vi "Report Options.vi"(5 "LensList":i32[](array[numeric]), 6 "Search Window":dbl=3.0 min=0.1 format="%#.6f", 7 "Min. Height":dbl=1.0 min=1.0 format="%#.6f", 8 "Min. Width":i32=4 min=2 max=100, 9 "RefMass":dbl[](array[numeric])) -> (0 "Search Window 2":dbl=3.0 min=0.1 format="%#.6f", 1 "Min. Height 2":dbl=1.0 min=1.0 format="%#.6f", 2 "Min. Width 2":i32=4 min=2 max=100, 3 "RefMass 2":dbl[](array[numeric]), 4 "LensList 2":i32[](array[numeric]))   [LabVIEW 2012]
uses:
  Configuration/_Global Configuration.vi
  <vilib>/Utility/file.llb/Read From Spreadsheet File (DBL).vi
  <vilib>/Utility/file.llb/Write To Spreadsheet File (DBL).vi
  <vilib>/Utility/config.llb/Write Key (String).vi
  <vilib>/Utility/config.llb/Write Key (Double).vi
  <vilib>/Utility/config.llb/Write Key (I32).vi
  <vilib>/Utility/config.llb/NI_LVConfig.lvlib
panel:
  in  "Tab Control":enum32{"Lens Selection", "Peak List Options"}(tab)
  in  "Delete":bool
  in  "Insert":bool
  in  "Current Lens":u16(ring)
  in  "Lens Values":i32(listbox)
  in  "Save":bool
  in  "Load":bool
  in  "Current Reference":dbl=500.0 min=0.0 max=3000.0 format="%#.2f"
  in  "Insert 2":bool
  in  "Delete 2":bool
  in  "Mass Reference (amu)":i32(listbox)
  # "Peak Parameter"
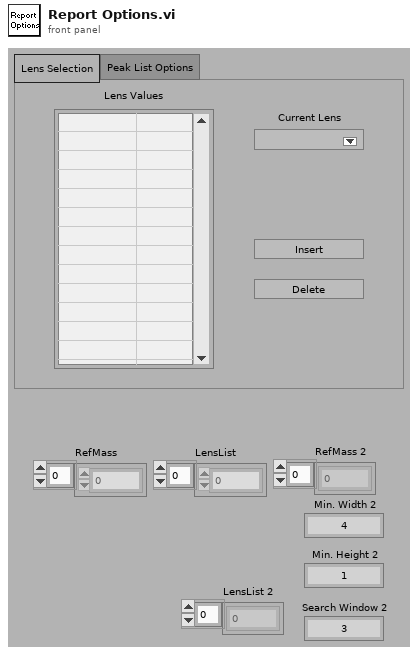
[diagram p1: front panel]
types:
  T1 = enum32{"existing file", "new file", "new or existing file", "existing dir", "new dir", "new or existing dir", "existing file (use LLBs)", "new file (use LLBs)", "new or existing file (use LLBs)", "new or existing file or directory (use LLBs)"}
  T2 = typedef "_RT Instrument 2.ctl" = cluster{"Table":T3[], "Instrument":string[]}
  T3 = typedef "_RT Configuration 2.ctl" = cluster{"Name":string, "Ch#":u8, "Min":dbl, "Max":dbl, "Def+":dbl, "Def-":dbl, "Offset":dbl, "Slope":dbl, "Type":u8, "Description":string, "SettleT":dbl}
  T4 = typedef "NI_LVConfig.lvlib/Config Data RefNum.ctl" = refnum<k1>
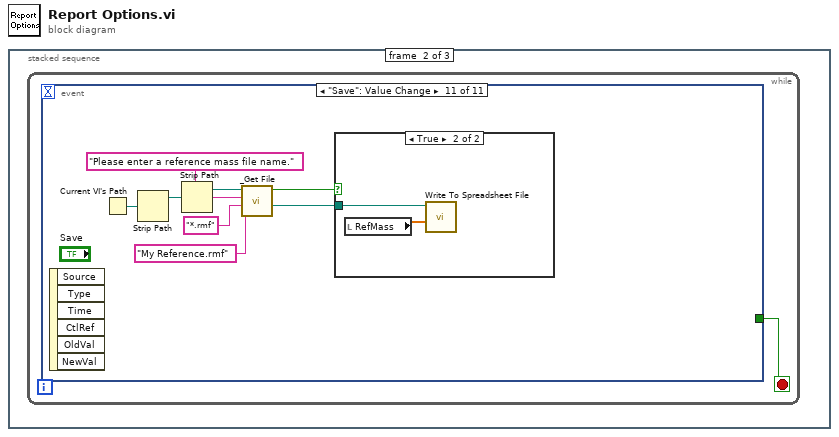
[diagram p0: block diagram]
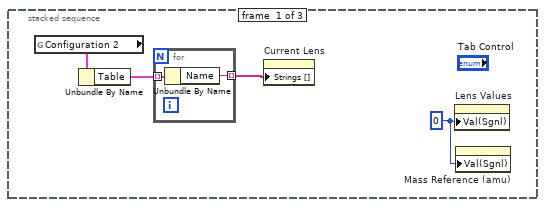
[diagram p2: hidden frame]
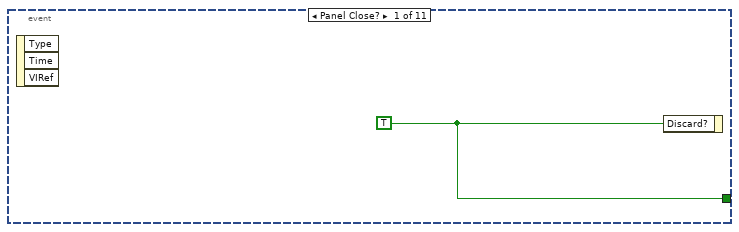
[diagram p3: hidden frame]
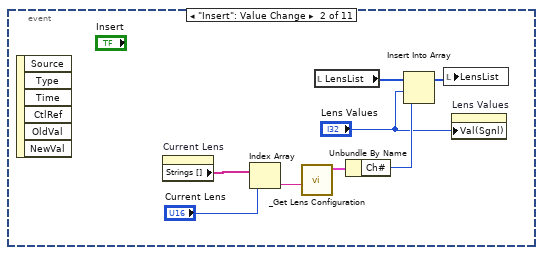
[diagram p4: hidden frame]
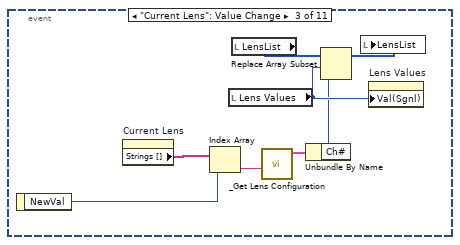
[diagram p5: hidden frame]
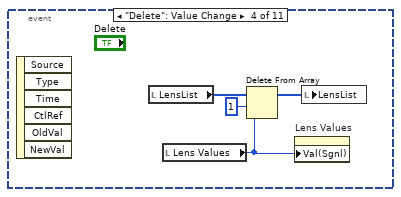
[diagram p6: hidden frame]
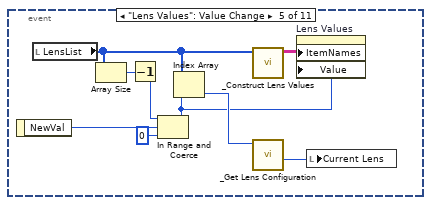
[diagram p7: hidden frame]
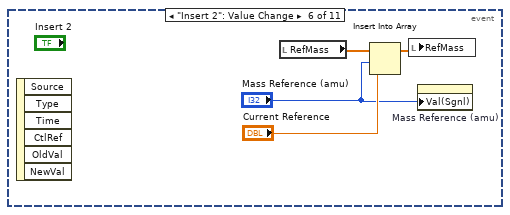
[diagram p8: hidden frame]
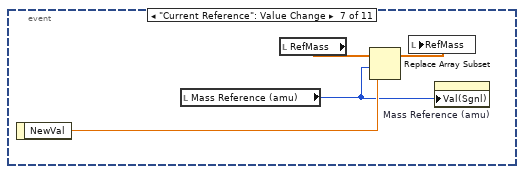
[diagram p9: hidden frame]
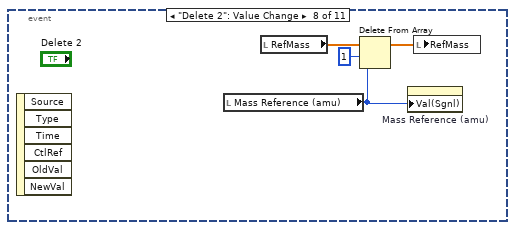
[diagram p10: hidden frame]
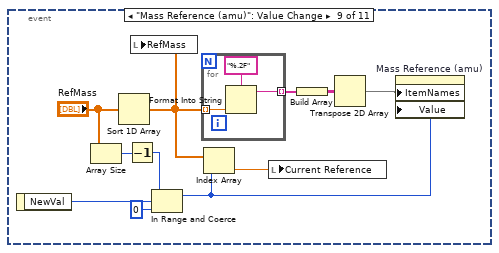
[diagram p11: hidden frame]
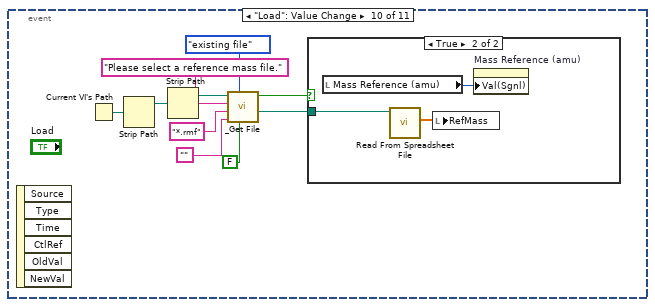
[diagram p12: hidden frame]
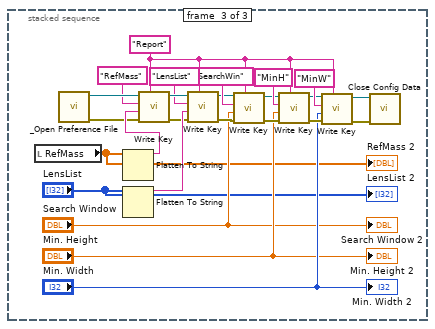
[diagram p15: hidden frame]
diagram:
  n1 = stacked-sequence {
    frame #0 {
      w1 = 0 ("Value (Signaling)")
      n2 = global read "_Global Configuration.vi" "Configuration 2"() -> (w3:T2)
      n3 = Unbundle By Name(w3) -> ("Table"=w2:T3[])
      n4 = for {
        tunnel: w2 -> [w6] mode=indexing
        tunnel: [w5] -> w4 mode=indexing
        n5 = Unbundle By Name(w6) -> ("Name"=w5:string)
      }
      n6 = property on="Current Lens" class="Ring (strict)"("Strings []"=w4) -> ()  [unwired: 2 in, 2 out]
      n7 = property on="Lens Values" class="MCListbox (strict)"("Val(Sgnl)"=w1) -> ()  [unwired: 2 in, 2 out]
      n8 = property on="Mass Reference (amu)" class="MCListbox (strict)"("Val(Sgnl)"=w1) -> ()  [unwired: 2 in, 2 out]
    }
    frame #1 {
      n9 = while {
        stop <- w7 stop-if-true
        n10 = event shown="[10] \"Save\": Value Change" {
          selector: _ -> [_ _ _ _ _ _ _ _ _ _ _]
          dyn-events: _ -> [_ _ _ _ _ _ _ _ _ _ _]
          timeout: _ -> [_ _ _ _ _ _ _ _ _ _ _]
          tunnel: [w8 _ _ _ _ _ _ _ _ _ _] -> w7
          event Panel Close? {
            w8 = TRUE ("Discard?")
            n11 = event-data() -> ()  [unwired: 4 out]
            n12 = event-data("Discard?"=w8) -> ()  [unwired: 1 in, 1 out]
          }
          event "Insert": Value Change {
            n13 = event-data() -> ()  [unwired: 7 out]
            n14 = property on="Current Lens" class="Ring (strict)"() -> ("Strings []"=w16:string[])  [unwired: 2 in, 2 out]
            n15 = Index Array(array=w16, index="Current Lens") -> (element=w14:string)
            n16 = call "_Get Lens Configuration.vi"("Name"=w14) -> ("Lens Configuration"=w13:T3)  [unwired: 1 in, 5 out]
            n17 = local read "LensList"() -> (w12:i32[])
            n18 = Unbundle By Name(w13) -> ("Ch#"=w11:u8)
            n19 = Insert Into Array(array=w12, index="Lens Values", new element=w11) -> (w10:i32[])
            n20 = local write "LensList"(w10) -> ()
            n21 = property on="Lens Values" class="MCListbox (strict)"("Val(Sgnl)"="Lens Values") -> ()  [unwired: 2 in, 2 out]
          }
          event "Current Lens": Value Change {
            n22 = event-data() -> ("NewVal"=w18:u16)  [unwired: 1 out]
            n23 = property on="Current Lens" class="Ring (strict)"() -> ("Strings []"=w20:string[])  [unwired: 2 in, 2 out]
            n24 = Index Array(array=w20, index=w18) -> (element=w21:string)
            n25 = local read "Lens Values"() -> (w24:i32)
            n26 = local read "LensList"() -> (w23:i32[])
            n27 = call "_Get Lens Configuration.vi"("Name"=w21) -> ("Lens Configuration"=w19:T3)  [unwired: 1 in, 5 out]
            n28 = Unbundle By Name(w19) -> ("Ch#"=w17:u8)
            n29 = Replace Array Subset(array=w23, new element=w17, index=w24) -> (w22:i32[])
            n30 = local write "LensList"(w22) -> ()
            n31 = property on="Lens Values" class="MCListbox (strict)"("Val(Sgnl)"=w24) -> ()  [unwired: 2 in, 2 out]
          }
          event "Delete": Value Change {
            n32 = event-data() -> ()  [unwired: 7 out]
            n33 = local read "LensList"() -> (w27:i32[])
            n34 = local read "Lens Values"() -> (w25:i32)
            n35 = Delete From Array(array=w27, length=1, index=w25) -> (array with subset deleted=w26:i32[])  [unwired: 1 out]
            n36 = property on="Lens Values" class="MCListbox (strict)"("Val(Sgnl)"=w25) -> ()  [unwired: 2 in, 2 out]
            n37 = local write "LensList"(w26) -> ()
          }
          event "Lens Values": Value Change {
            n38 = event-data() -> ("NewVal"=w32:i32)  [unwired: 1 out]
            n39 = local read "LensList"() -> (w34:i32[])
            n40 = Array Size(array=w34) -> (size(s)=w33:i32)
            n41 = Decrement(x=w33) -> (x-1=w31:i32)
            n42 = In Range and Coerce(upper limit=w31, x=w32, lower limit=0) -> (coerced(x)=w29:i32)  [unwired: 1 out]
            n43 = Index Array(array=w34, index=w29) -> (element=w37:i32)
            n44 = call "_Construct Lens Values.vi"("Lens List"=w34) -> ("Table"=w35:string[][])  [unwired: 6 out]
            n45 = call "_Get Lens Configuration.vi"("Channel #"=w37) -> ("Config Row#"=w36:i32)  [unwired: 1 in, 5 out]
            n46 = property on="Lens Values" class="MCListbox (strict)"("ItemNames"=w35, "Value"=w29) -> ()  [unwired: 2 in, 2 out]
            n47 = local write "Current Lens"(w36) -> ()
          }
          event "Insert 2": Value Change {
            n48 = event-data() -> ()  [unwired: 7 out]
            n49 = local read "RefMass"() -> (w39:dbl[])
            n50 = Insert Into Array(array=w39, index="Mass Reference (amu)", new element="Current Reference") -> (w38:dbl[])
            n51 = local write "RefMass"(w38) -> ()
            n52 = property on="Mass Reference (amu)" class="MCListbox (strict)"("Val(Sgnl)"="Mass Reference (amu)") -> ()  [unwired: 2 in, 2 out]
          }
          event "Current Reference": Value Change {
            n53 = event-data() -> ("NewVal"=w43:dbl)  [unwired: 1 out]
            n54 = local read "Mass Reference (amu)"() -> (w42:i32)
            n55 = local read "RefMass"() -> (w45:dbl[])
            n56 = Replace Array Subset(array=w45, new element=w43, index=w42) -> (w44:dbl[])
            n57 = local write "RefMass"(w44) -> ()
            n58 = property on="Mass Reference (amu)" class="MCListbox (strict)"("Val(Sgnl)"=w42) -> ()  [unwired: 2 in, 2 out]
          }
          event "Delete 2": Value Change {
            n59 = event-data() -> ()  [unwired: 7 out]
            n60 = local read "Mass Reference (amu)"() -> (w46:i32)
            n61 = local read "RefMass"() -> (w48:dbl[])
            n62 = Delete From Array(array=w48, length=1, index=w46) -> (array with subset deleted=w47:dbl[])  [unwired: 1 out]
            n63 = property on="Mass Reference (amu)" class="MCListbox (strict)"("Val(Sgnl)"=w46) -> ()  [unwired: 2 in, 2 out]
            n64 = local write "RefMass"(w47) -> ()
          }
          event "Mass Reference (amu)": Value Change {
            n65 = event-data() -> ("NewVal"=w57:i32)  [unwired: 1 out]
            n66 = Array Size(array="RefMass") -> (size(s)=w54:i32)
            n67 = Sort 1D Array(array="RefMass") -> (sorted array=w50:dbl[])
            n68 = Decrement(x=w54) -> (x-1=w53:i32)
            n69 = local write "RefMass"(w50) -> ()
            n70 = In Range and Coerce(upper limit=w53, x=w57, lower limit=0) -> (coerced(x)=w51:i32)  [unwired: 1 out]
            n71 = for {
              tunnel: w50 -> [w63] mode=indexing
              tunnel: [w61] -> w59 mode=indexing
              n72 = Format Into String(format string="%.2F", w63) -> (resulting string=w61:string)  [unwired: 2 in, 1 out]
            }
            n73 = Index Array(array=w50, index=w51) -> (element=w58:dbl)
            n74 = local write "Current Reference"(w58) -> ()
            n75 = Build Array(w59) -> (w60:string[][])
            n76 = Transpose 2D Array(2D array=w60) -> (transposed array=w52:string[][])
            n77 = property on="Mass Reference (amu)" class="MCListbox (strict)"("ItemNames"=w52, "Value"=w51) -> ()  [unwired: 2 in, 2 out]
          }
          event "Load": Value Change {
            n78 = event-data() -> ()  [unwired: 7 out]
            n79 = Current VI's Path() -> (path=w73:path)
            n80 = Strip Path(path=w73) -> (stripped path=w72:path)  [unwired: 1 out]
            n81 = Strip Path(path=w72) -> (stripped path=w71:path)  [unwired: 1 out]
            n82 = call "_Get File.vi"("For Write (T)"=FALSE, "select mode (new or existing)"=T1."existing file", "default name"="", "extension (isd)"="*.rmf", "prompt"="Please select a reference mass file.", "Start Path"=w71) -> ("Seleted File"=w67:path, "Succeeded"=w68:bool)  [unwired: 2 out]
            n83 = case shown="True" w68 {
              tunnel: w67 -> [_ w76]
              frame False {
              }
              frame True {
                n84 = local read "Mass Reference (amu)"() -> (w74:i32)
                n85 = call-poly <vilib>:"Read From Spreadsheet File.vi"("file path (dialog if empty)"=w76) -> ("first row"=w75:dbl[])  [unwired: 3 in, 7 out]
                n86 = local write "RefMass"(w75) -> ()
                n87 = property on="Mass Reference (amu)" class="MCListbox (strict)"("Val(Sgnl)"=w74) -> ()  [unwired: 2 in, 2 out]
              }
            }
          }
          event "Save": Value Change {
            n88 = event-data() -> ()  [unwired: 7 out]
            n89 = Current VI's Path() -> (path=w84:path)
            n90 = Strip Path(path=w84) -> (stripped path=w83:path)  [unwired: 1 out]
            n91 = Strip Path(path=w83) -> (stripped path=w82:path)  [unwired: 1 out]
            n92 = call "_Get File.vi"("default name"="My Reference.rmf", "extension (isd)"="*.rmf", "prompt"="Please enter a reference mass file name.", "Start Path"=w82) -> ("Seleted File"=w78:path, "Succeeded"=w79:bool)  [unwired: 2 in, 2 out]
            n93 = case shown="True" w79 {
              tunnel: w78 -> [_ w86]
              frame False {
              }
              frame True {
                n94 = local read "RefMass"() -> (w85:dbl[])
                n95 = call-poly <vilib>:"Write To Spreadsheet File.vi"("1D data"=w85, "file path (dialog if empty)"=w86) -> ()  [unwired: 4 in, 3 out]
              }
            }
          }
        }
      }
    }
    frame #2 {
      w101 = "Report" ("section")
      n96 = local read "RefMass"() -> (w87:dbl[])
      "RefMass 2" <- w87
      n97 = call "_Open Preference File.vi"() -> ("error"=w97:errorcluster, "refnum"=w109:T4)  [unwired: 1 in, 5 out]
      n98 = Flatten To String(anything=w87) -> (data string=w98:string)  [unwired: 1 in, 4 out]
      n99 = Flatten To String(anything="LensList") -> (data string=w96:string)  [unwired: 1 in, 4 out]
      n100 = call-poly <vilib>:"Write Key.vi"("section"=w101, "error in (no error)"=w97, "value"=w98, "key"="RefMass", "refnum"=w109) -> ("error out"=w95:errorcluster, "refnum out"=w111:T4)  [unwired: 1 in, 4 out]
      n101 = call-poly <vilib>:"Write Key.vi"("section"=w101, "error in (no error)"=w95, "value"=w96, "key"="LensList" ("section"), "refnum"=w111) -> ("error out"=w94:errorcluster, "refnum out"=w104:T4)  [unwired: 1 in, 4 out]
      n102 = call-poly <vilib>:"Write Key.vi"("section"=w101, "error in (no error)"=w94, "value"="Search Window", "key"="SearchWin", "refnum"=w104) -> ("error out"=w93:errorcluster, "refnum out"=w105:T4)  [unwired: 3 in, 2 out]
      n103 = call-poly <vilib>:"Write Key.vi"("section"=w101, "error in (no error)"=w93, "value"="Min. Height", "key"="MinH" ("section"), "refnum"=w105) -> ("error out"=w92:errorcluster, "refnum out"=w102:T4)  [unwired: 3 in, 2 out]
      n104 = call-poly <vilib>:"Write Key.vi"("section"=w101, "error in (no error)"=w92, "value"="Min. Width", "key"="MinW" ("section"), "refnum"=w102) -> ("error out"=w99:errorcluster, "refnum out"=w100:T4)  [unwired: 5 out]
      n105 = call <vilib>:"Close Config Data.vi"("error in (no error)"=w99, "refnum"=w100) -> ()  [unwired: 1 in, 9 out]
      "Min. Width 2" <- "Min. Width"
      "Min. Height 2" <- "Min. Height"
      "Search Window 2" <- "Search Window"
      "LensList 2" <- "LensList"
    }
  }
